vi "TrafficLight.vi"() -> ()   [LabVIEW 2015]
panel:
  out "Numeric 3":dbl
  in  "Conditions":T1(radio)
  out "Boolean":bool
  in  "Numeric":dbl=1.0 min=1.0 max=6.0
  in  "stop":bool
  out "Green NS":bool
  out "Yellow NS":bool
  out "Red NS":bool
  out "Green WE":bool
  out "Yellow WE":bool
  out "Red WE":bool
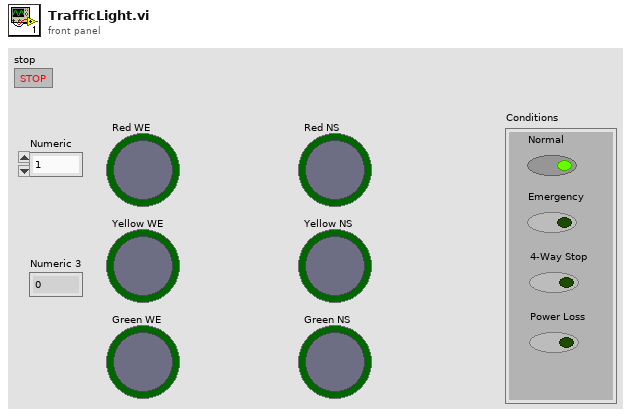
[diagram p1: front panel]
types:
  T1 = enum32{"Normal", "Emergency", "4-Way Stop", "Power Loss"}
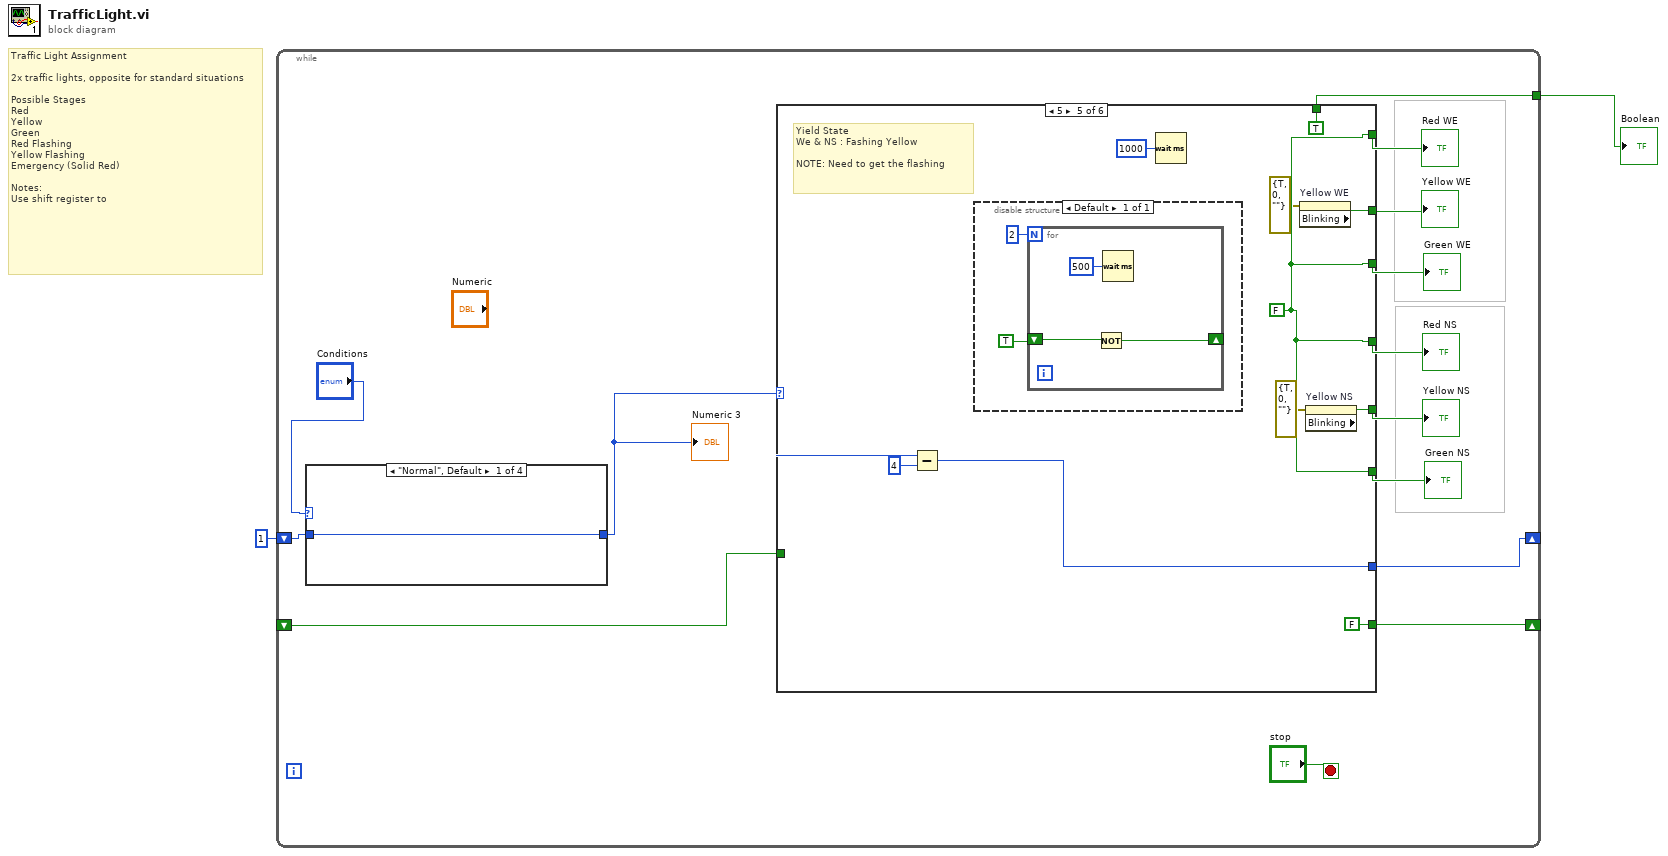
[diagram p0: block diagram]
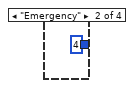
[diagram p2: hidden frame]
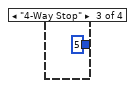
[diagram p3: hidden frame]
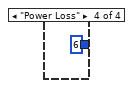
[diagram p4: hidden frame]
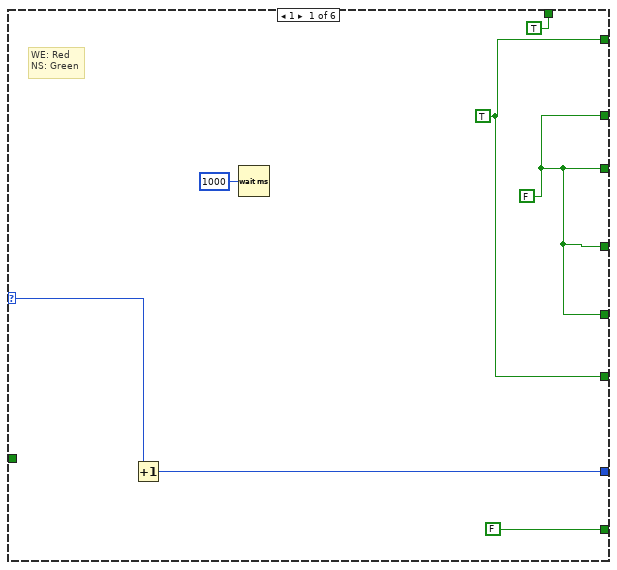
[diagram p5: hidden frame]
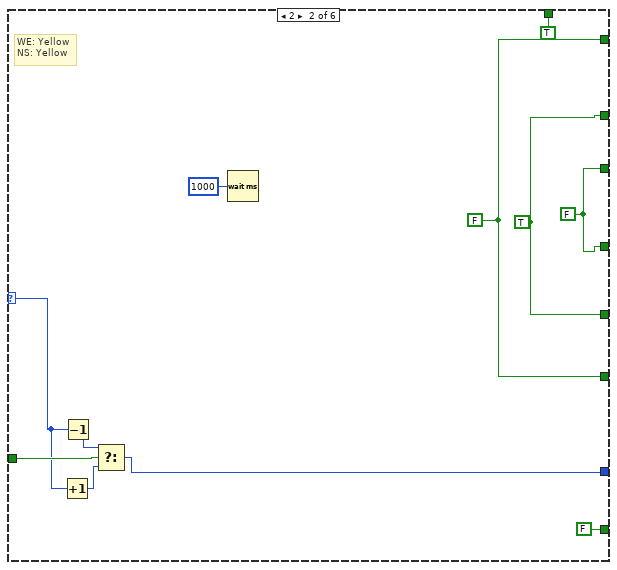
[diagram p6: hidden frame]
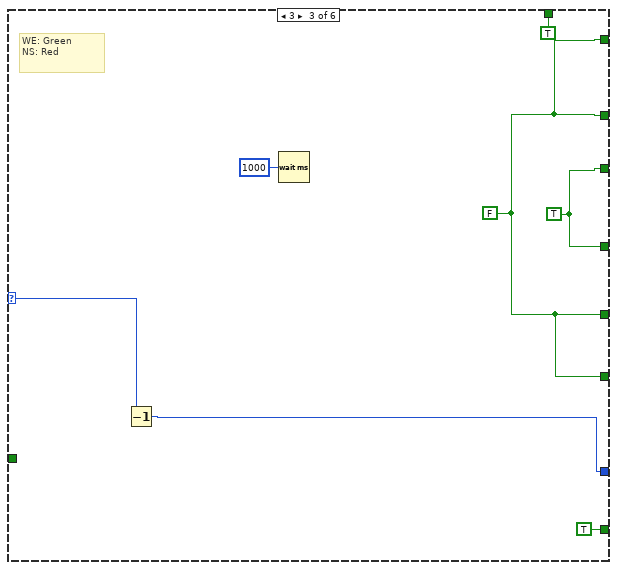
[diagram p7: hidden frame]
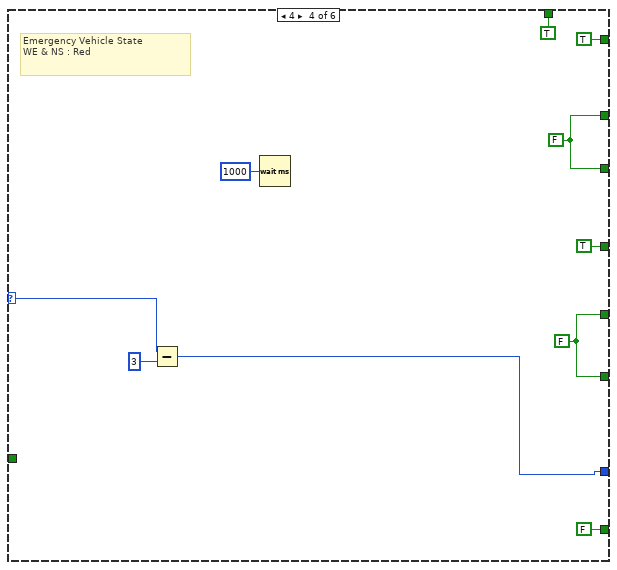
[diagram p8: hidden frame]
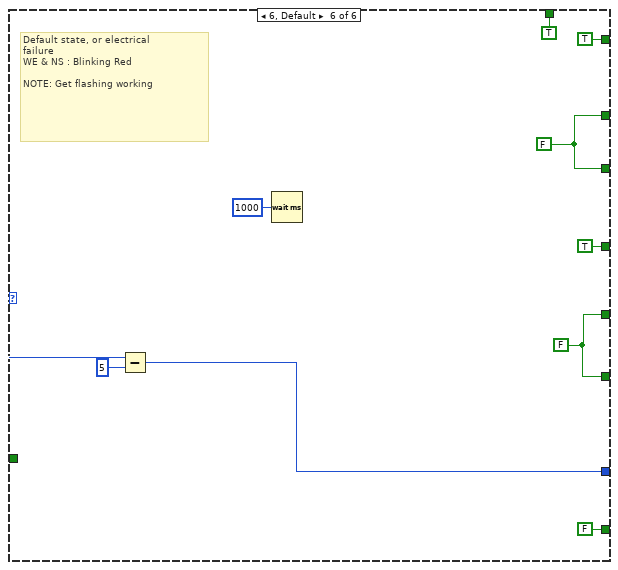
[diagram p9: hidden frame]
diagram:
  # "Traffic Light Assignment\n\n2x traffic lights, opposite for standard situations\n\nPossible Stages\nRed\nYellow\nGreen\nRed Flashing\nYellow Flashing\nEmergency (Solid Red)\n\nNotes:\nUse shift register to"
  n1 = while {
    tunnel: [w9] -> w2
    shift-right: [w8] -> _
    shift-left: 1 -> [w5]
    shift-right: [w4] -> _
    shift-left: _ -> [w3]
    stop <- "stop" stop-if-true
    n2 = case shown="\"Normal\", Default" "Conditions" {
      tunnel: [w17 4 5 6] -> w7
      tunnel: w5 -> [w17 _ _ _]
      frame "Normal", Default {
      }
      frame "Emergency" {
      }
      frame "4-Way Stop" {
      }
      frame "Power Loss" {
      }
    }
    "Numeric 3" <- w7
    n3 = case shown="5" w7 {
      selector: w7 -> [w24 w28 w41 w49 w63 w75]
      tunnel: [w27 w37 w45 w53 w66 w79] -> w15
      tunnel: [w27 w38 w44 w53 w59 w79] -> w14
      tunnel: [w26 w36 w44 TRUE w66 TRUE] -> w13
      tunnel: [w27 w37 w45 TRUE w66 TRUE] -> w12
      tunnel: [w27 w38 w44 w52 w57 w78] -> w11
      tunnel: [w26 w36 w44 w52 w66 w78] -> w10
      tunnel: [TRUE ("Boolean") TRUE ("Boolean") TRUE ("Boolean") TRUE ("Boolean") TRUE ("Boolean") TRUE ("Boolean")] -> w9
      tunnel: [w23 w31 w40 w47 w61 w73] -> w8
      tunnel: [FALSE FALSE TRUE FALSE FALSE FALSE] -> w4
      tunnel: w3 -> [_ w32 _ _ _ _]
      frame 1 {
        w26 = TRUE
        w27 = FALSE
        # "WE: Red\nNS: Green"
        n4 = Increment(x=w24) -> (x+1=w23:i32)
        n5 = Wait (ms)(milliseconds to wait=u32 1000) -> ()  [unwired: 1 out]
      }
      frame 2 {
        w36 = FALSE
        w37 = FALSE
        w38 = TRUE
        # "WE: Yellow\nNS: Yellow"
        n6 = Increment(x=w28) -> (x+1=w29:i32)
        n7 = Decrement(x=w28) -> (x-1=w30:i32)
        n8 = Select(t=w30, s=w32, f=w29) -> (s? t:f=w31:i32)
        n9 = Wait (ms)(milliseconds to wait=u32 1000) -> ()  [unwired: 1 out]
      }
      frame 3 {
        w44 = FALSE
        w45 = TRUE
        # "WE: Green\nNS: Red"
        n10 = Decrement(x=w41) -> (x-1=w40:i32)
        n11 = Wait (ms)(milliseconds to wait=u32 1000) -> ()  [unwired: 1 out]
      }
      frame 4 {
        w52 = FALSE
        w53 = FALSE
        # "Emergency Vehicle State\nWE & NS : Red"
        n12 = Subtract(x=w49, y=3) -> (x-y=w47:i32)
        n13 = Wait (ms)(milliseconds to wait=u32 1000) -> ()  [unwired: 1 out]
      }
      frame 5 {
        w66 = FALSE
        # "Yield State\nWe & NS : Fashing Yellow\n\nNOTE: Need to get the flashing"
        n14 = Subtract(x=w63, y=4) -> (x-y=w61:i32)
        n15 = disable-structure shown="Default" {
          frame Enabled {
            n16 = for {
              N: 2 -> [_]
              shift-right: [w70] -> _
              shift-left: TRUE -> [w71]
              n17 = Not(x=w71) -> (.not. x?=w70:bool)
              n18 = Wait (ms)(milliseconds to wait=u32 500) -> ()  [unwired: 1 out]
            }
          }
        }
        n19 = Wait (ms)(milliseconds to wait=u32 1000) -> ()  [unwired: 1 out]
        n20 = property on="Yellow WE" class="Bool (strict)"(error in=errorcluster {"status"=TRUE, "code"=0, "source"=""} ("error in (no error)")) -> ("Blinking"=w59:bool)  [unwired: 1 in, 2 out]
        n21 = property on="Yellow NS" class="Bool (strict)"(error in=errorcluster {"status"=TRUE, "code"=0, "source"=""} ("error in (no error)")) -> ("Blinking"=w57:bool)  [unwired: 1 in, 2 out]
      }
      frame 6, Default {
        w78 = FALSE
        w79 = FALSE
        # "Default state, or electrical\nfailure\nWE & NS : Blinking Red\n\nNOTE: Get flashing working"
        n22 = Subtract(x=w75, y=5) -> (x-y=w73:i32)
        n23 = Wait (ms)(milliseconds to wait=u32 1000) -> ()  [unwired: 1 out]
      }
    }
    "Red NS" <- w12
    "Yellow NS" <- w11
    "Green NS" <- w10
    "Red WE" <- w13
    "Yellow WE" <- w14
    "Green WE" <- w15
  }
  "Boolean" <- w2
